vi "Kinect Global.vi"() -> ()   [LabVIEW 2014]
uses:
  Resources/Others/Control cluster.ctl
panel:
  out "Control Cluster":T1={"Roll"=-0.03, "Pitch"=-0.052222222, "Vertical Speed"=0.0, "Yaw Speed"=0.0} {"Yaw Speed" scale=-1.0..1.0; "Vertical Speed" scale=-1.0..1.0; "Pitch" scale=-1.0..1.0; "Roll" scale=-1.0..1.0}
  in  "Weak detection":bool
  in  "Hover":bool
  in  "Toggle Land/Take off":bool
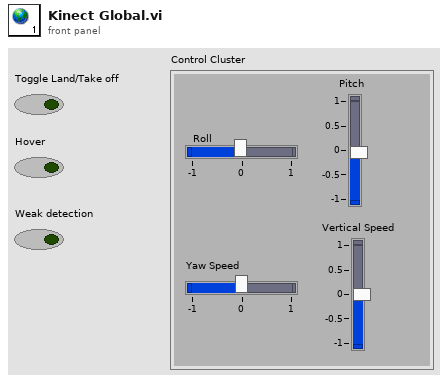
[diagram p1: front panel]
types:
  T1 = typedef "Control cluster.ctl" = cluster{"Roll":sgl, "Pitch":sgl, "Vertical Speed":sgl, "Yaw Speed":sgl}
diagram:
